vi "Viavi - Single Channel Table.vi"(11 "Data Input":T2) -> (3 "Table Output":T1(array[cluster]))   [LabVIEW 2017]
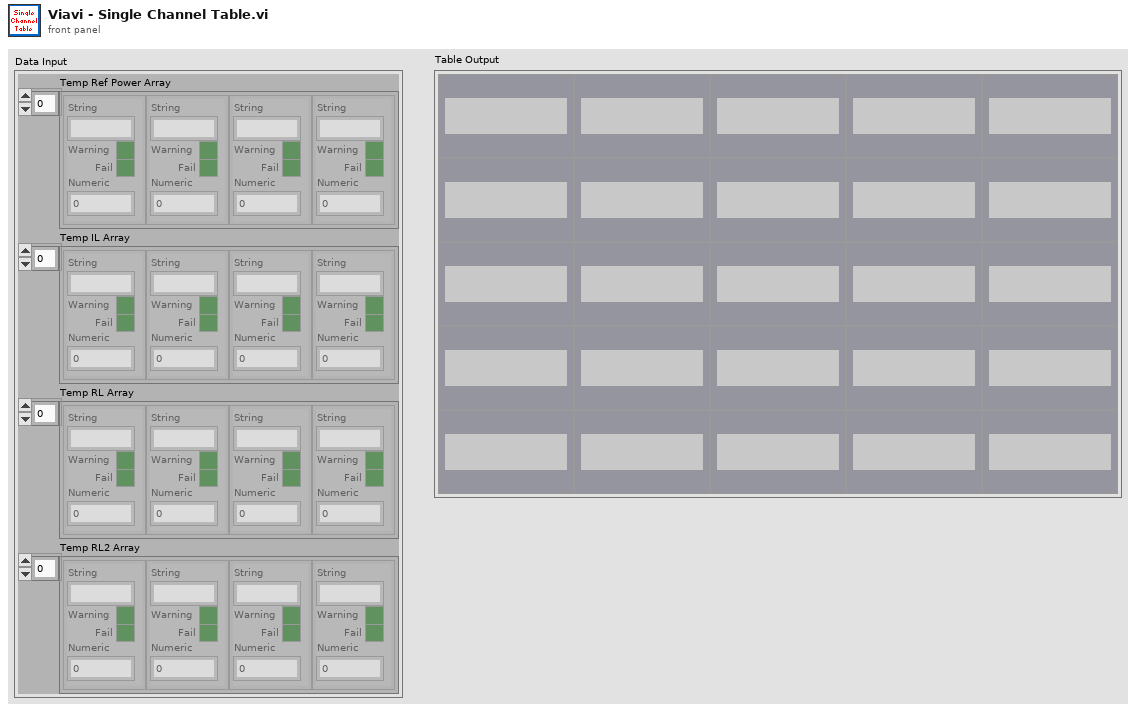
[diagram p1: front panel]
types:
  T1 = cluster{"String":string, "Warning":bool, "Fail":bool, "Numeric":dbl}[][]
  T2 = cluster{"Temp Ref Power Array":cluster{"String":string, "Warning":bool, "Fail":bool, "Numeric":dbl}[], "Temp IL Array":cluster{"String":string, "Warning":bool, "Fail":bool, "Numeric":dbl}[], "Temp RL Array":cluster{"String":string, "Warning":bool, "Fail":bool, "Numeric":dbl}[], "Temp RL2 Array":cluster{"String":string, "Warning":bool, "Fail":bool, "Numeric":dbl}[]}
  T3 = cluster{"String":string, "Warning":bool, "Fail":bool, "Numeric":dbl}[]
  T4 = cluster{"String":string, "Warning":bool, "Fail":bool, "Numeric":dbl}
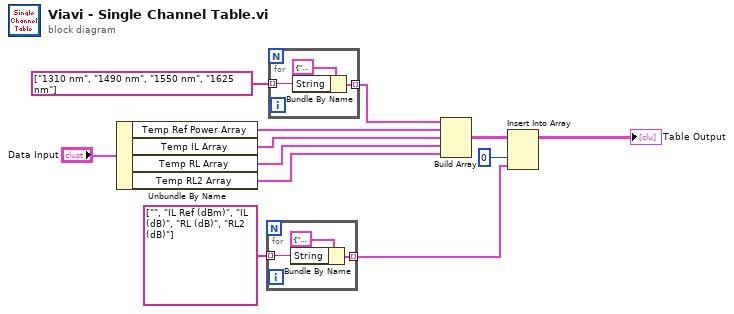
[diagram p0: block diagram]
diagram:
  n1 = Unbundle By Name("Data Input") -> ("Temp Ref Power Array"=w9:T3, "Temp IL Array"=w8:T3, "Temp RL Array"=w7:T3, "Temp RL2 Array"=w6:T3)
  n2 = for {
    tunnel: string[] ["", "IL Ref (dBm)", "IL (dB)", "RL (dB)", "RL2 (dB)"] -> [w14] mode=indexing
    tunnel: [w13] -> w4 mode=indexing
    n3 = Bundle By Name(cluster=T4 {"String"="", "Warning"=FALSE, "Fail"=FALSE, "Numeric"=0.0} ("Single Cell Cluster"), "String"=w14) -> (w13:T4)
  }
  n4 = for {
    tunnel: string[] ["1310 nm", "1490 nm", "1550 nm", "1625 nm"] -> [w17] mode=indexing
    tunnel: [w16] -> w2 mode=indexing
    n5 = Bundle By Name(cluster=T4 {"String"="", "Warning"=FALSE, "Fail"=FALSE, "Numeric"=0.0} ("Single Cell Cluster"), "String"=w17) -> (w16:T4)
  }
  n6 = Build Array(w2, w9, w8, w7, w6) -> (w12:T1)
  n7 = Insert Into Array(array=w12, index (col)=0 ("index (row)"), new element=w4) -> (→"Table Output":T1)  [unwired: 1 in]
